vi "Flatten.vi"(8 "error in":errorcluster, 9 "Data":T1) -> (0 "error out":errorcluster, 2 "Buffer":u8[](array[numeric]) format="%.0x")   [LabVIEW 2020, in "TcpAckNack.lvlib"]
uses:
  TcpAckNack.lvlib
  lv-protoc/LV-Proto/LV-Proto.lvlib
  AckNackResult/AckNackResult.lvlib
  Data.ctl
  AckNackResult/Enumeration.ctl
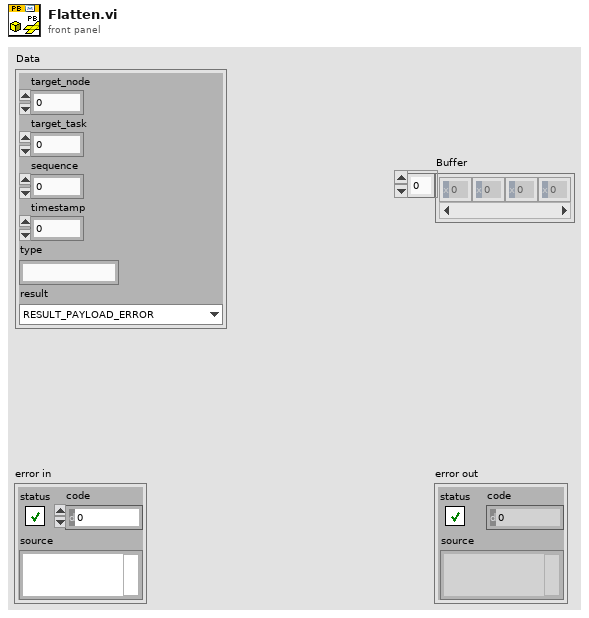
[diagram p1: front panel]
types:
  T1 = typedef "TcpAckNack.lvlib/Data.ctl" = cluster{"target_node":u32, "target_task":u32, "sequence":u32, "timestamp":u64, "type":string, "result":T2}
  T2 = typedef "AckNackResult.lvlib/Enumeration.ctl" = enum16{"RESULT_PAYLOAD_ERROR", "RESULT_UNEXPECTED_TYPE", "RESULT_EXPIRED", "RESULT_OUTOFSEQUENCE", "RESULT_DISALLOWED", "RESULT_INVALIDTASK", "RESULT_INVALIDTARGET", "RESULT_UNKNOWN", "RESULT_ACK"}
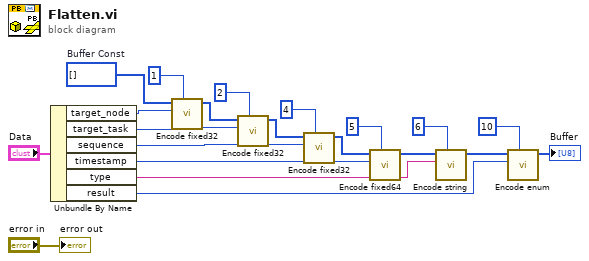
[diagram p0: block diagram]
diagram:
  w19 = u8[] []  # Buffer Const
  n1 = Unbundle By Name("Data") -> ("target_node"=w17:u32, "target_task"=w14:u32, "sequence"=w11:u32, "timestamp"=w8:u64, "type"=w5:string, "result"=w2:T2)
  n2 = call "Encode fixed32.vi"("Field Number"=1, "fixed32"=w17, "Buffer in"=w19) -> ("Buffer"=w16:u8[])  [unwired: 8 in]
  n3 = call "Encode fixed32.vi"("Field Number"=2, "fixed32"=w14, "Buffer in"=w16) -> ("Buffer"=w13:u8[])  [unwired: 8 in]
  n4 = call "Encode fixed32.vi"("Field Number"=4, "fixed32"=w11, "Buffer in"=w13) -> ("Buffer"=w10:u8[])  [unwired: 8 in]
  n5 = call "Encode fixed64.vi"("Field Number"=5, "fixed64"=w8, "Buffer in"=w10) -> ("Buffer"=w7:u8[])  [unwired: 8 in]
  n6 = call "Encode string.vi"("Field Number"=6, "string"=w5, "Buffer in"=w7) -> ("Buffer"=w4:u8[])  [unwired: 8 in]
  n7 = call "Encode enum.vi"("Field Number"=10, "Enumeration"=w2, "Buffer in"=w4) -> ("Buffer"=→"Buffer":u8[])  [unwired: 8 in]
  "error out" <- "error in"
